vi "Write current filename.vi"(8 "error in (no error)":errorcluster, 10 "current filename":path, 11 "Manage File Response in":refnum<class "Manage File Response.lvclass">) -> (0 "error out":errorcluster, 3 "Manage File Response out":refnum<class "Manage File Response.lvclass">)   [LabVIEW 2020, in "AIM ARINC 664 Engine.lvlib" / "Implementation.lvlib" / "Frame Logging.lvlib" / "Manage File Response.lvclass"]
uses:
  Manage File Response.lvclass
  Manage File Response.lvclass/Manage File Response.ctl
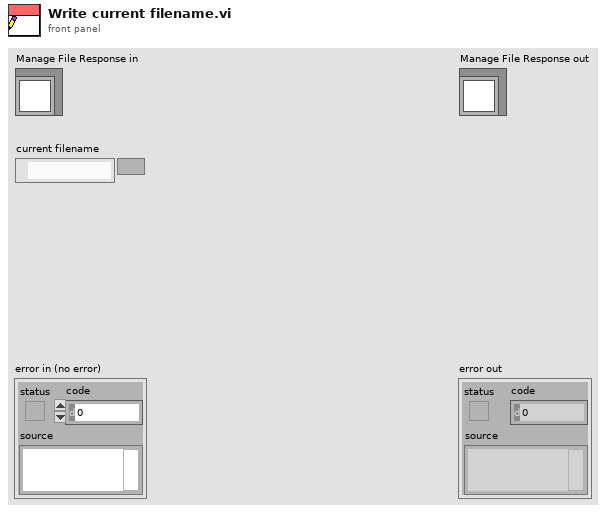
[diagram p1: front panel]
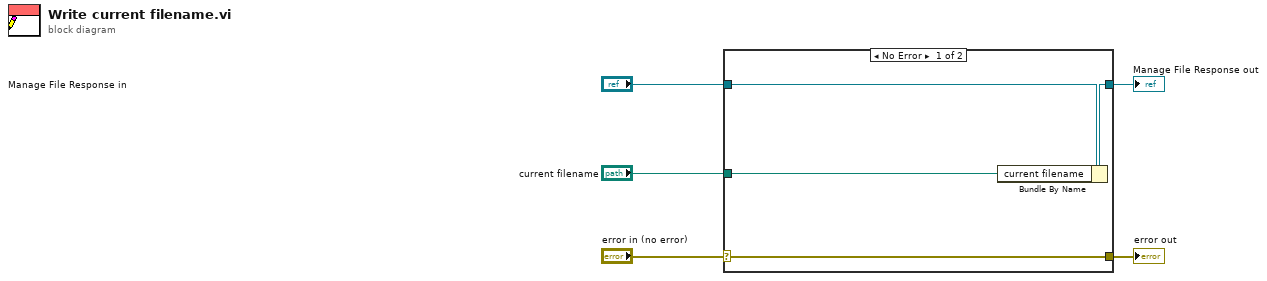
[diagram p0: block diagram]
diagram:
  n1 = case shown="No Error" "error in (no error)" {
    selector: "error in (no error)" -> [w9 w10]
    tunnel: [w9 w10] -> w4
    tunnel: [w7 w11] -> w2
    tunnel: "Manage File Response in" -> [w8 w11]
    tunnel: "current filename" -> [w6 _]
    frame No Error {
      n2 = Bundle By Name(cluster=w8, "current filename"=w6) -> (w7:refnum<class "Manage File Response.lvclass">)
    }
    frame Error {
    }
  }
  "error out" <- w4
  "Manage File Response out" <- w2
